vi "Actor Core.vi"(8 "error in":errorcluster, 11 "Chat Room Model in":refnum<class "Chat Room Model.lvclass">) -> (0 "error out":errorcluster, 3 "Actor out":refnum<class "Actor.lvclass">)   [LabVIEW 2025, in "Chat Room Model.lvlib" / "Chat Room Model.lvclass"]
doc: "<p>(<strong>Filename</strong>: <span class=\"dnl\">Actor Framework.lvlib:Actor.lvclass:Actor Core.vi</span>)</p>\n<p>Receives messages to the actor, reacts to them, and initiates any error handling that may shut the actor down.</p>\n<p>Descendant classes may override this VI to append parallel tasks for the actor to complete while it handles messages. Overrides use the <a href=\"nihelplauncher://docs/csh?context=lvcore_glang_udclass\">Call Parent Class Method</a> node.</p>"
uses:
  Chat Room Model.lvclass
  <vilib>/ActorFramework/Actor/Actor.lvclass
  Chat Room Model.lvclass/Chat Room Model.ctl
  Chat Window Panel/Chat Window Panel.lvclass
  C:/Users/lm2cc/Desktop/Interface Atuadores Labview/Chat Room/Chat Room Controller/Chat Room Controller/Chat Room Controller.lvclass
  C:/Program Files (x86)/National Instruments/LabVIEW 2025/vi.lib/ActorFramework/Actor/Actor.lvclass
  C:/Users/lm2cc/Desktop/Interface Atuadores Labview/Chat Room/Chat Window Panel/Chat Window Panel.lvclass
  C:/Users/lm2cc/Desktop/Interface Atuadores Labview/Chat Room/Chat Room Model/Chat Room Model/Chat Room Model.lvclass
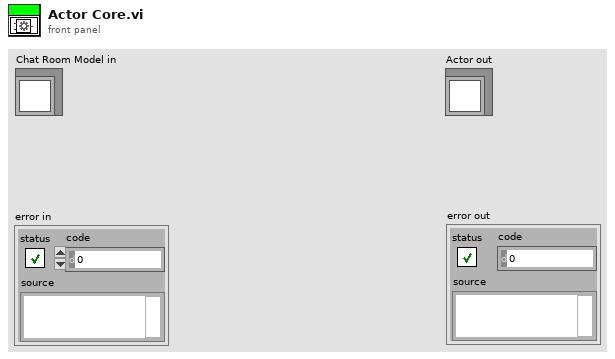
[diagram p1: front panel]
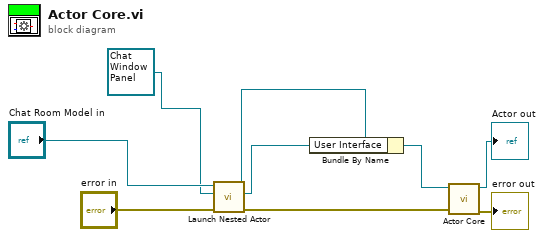
[diagram p0: block diagram]
diagram:
  n1 = call <vilib>:"Launch Nested Actor.vi"("error in (no error)"="error in", "Nested Actor"=refnum<class "Chat Window Panel.lvclass"> refnum ("Chat Window Panel.lvlib:Chat Window Panel.lvclass"), "Caller Actor in"="Chat Room Model in") -> ("error out"=w6:errorcluster, "Nested Actor's Enqueuer"=w4:refnum<class "Message Enqueuer.lvclass">, "Caller Actor in"=w2:refnum<class "Chat Room Model.lvclass">)  [unwired: 6 in]
  n2 = Bundle By Name(cluster=w2, "User Interface"=w4) -> (w3:refnum<class "Chat Room Model.lvclass">)
  n3 = call-parent "Actor Core.vi"("error in"=w6, "Actor in"=w3) -> ("error out"=→"error out":errorcluster, "Actor out"=→"Actor out":refnum<class "Actor.lvclass">)  [unwired: 8 in]
